vi "SubVI_ReadMatMask_001.vi"(0 "in IMG":bool[][](array[boolean])) -> (1 "Input current":i32[](array[numeric]), 2 "#iter":i32)   [LabVIEW 2018]
uses:
  <vilib>/Analysis/baseanly.llb/Real Dot Product.vi
  <vilib>/Analysis/NI_AALBase.lvlib
panel:
  out "mask":i16[][](array[numeric])
  out "in IMG":i16[][](array[numeric])
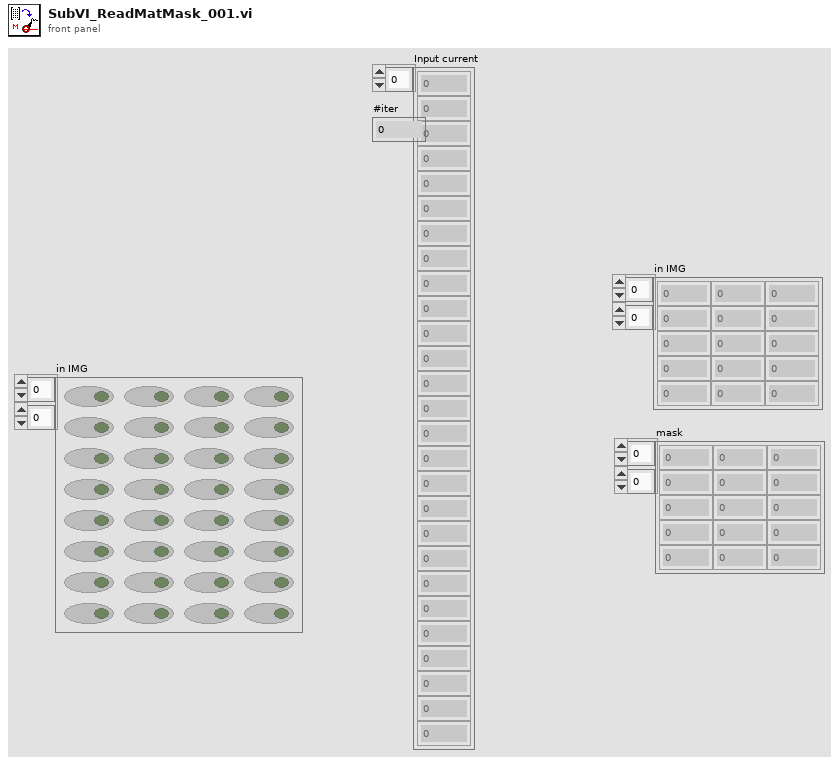
[diagram p1: front panel]
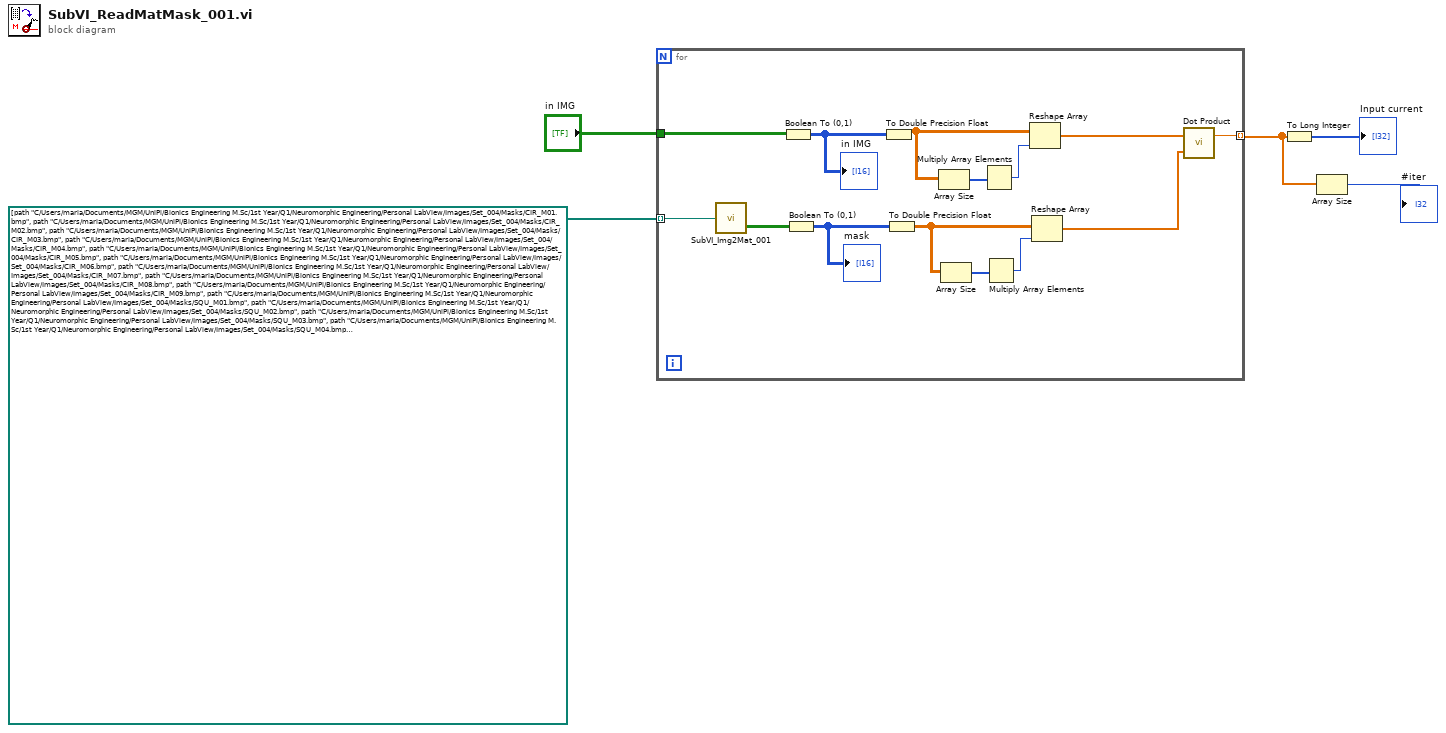
[diagram p0: block diagram]
diagram:
  n1 = for {
    tunnel: [w9] -> w2 mode=indexing
    tunnel: path[] [path "C:/Users/maria/Documents/MGM/UniPi/Bionics Engineering M.Sc/1st Year/Q1/Neuromorphic Engineering/Personal LabView/Images/Set_004/Masks/CIR_M01.bmp", path "C:/Users/maria/Documents/MGM/UniPi/Bionics Engineering M.Sc/1st Year/Q1/Neuromorphic Engineering/Personal LabView/Images/Set_004/Masks/CIR_M02.bmp", path "C:/Users/maria/Documents/MGM/UniPi/Bionics Engineering M.Sc/1st Year/Q1/Neuromorphic Engineering/Personal LabView/Images/Set_004/Masks/CIR_M03.bmp", path "C:/Users/maria/Documents/MGM/UniPi/Bionics Engineering M.Sc/1st Year/Q1/Neuromorphic Engineering/Personal LabView/Images/Set_004/Masks/CIR_M04.bmp", path "C:/Users/maria/Documents/MGM/UniPi/Bionics Engineering M.Sc/1st Year/Q1/Neuromorphic Engineering/Personal LabView/Images/Set_004/Masks/CIR_M05.bmp", path "C:/Users/maria/Documents/MGM/UniPi/Bionics Engineering M.Sc/1st Year/Q1/Neuromorphic Engineering/Personal LabView/Images/Set_004/Masks/CIR_M06.bmp", path "C:/Users/maria/Documents/MGM/UniPi/Bionics Engineering M.Sc/1st Year/Q1/Neuromorphic Engineering/Personal LabView/Images/Set_004/Masks/CIR_M07.bmp", path "C:/Users/maria/Documents/MGM/UniPi/Bionics Engineering M.Sc/1st Year/Q1/Neuromorphic Engineering/Personal LabView/Images/Set_004/Masks/CIR_M08.bmp", path "C:/Users/maria/Documents/MGM/UniPi/Bionics Engineering M.Sc/1st Year/Q1/Neuromorphic Engineering/Personal LabView/Images/Set_004/Masks/CIR_M09.bmp", path "C:/Users/maria/Documents/MGM/UniPi/Bionics Engineering M.Sc/1st Year/Q1/Neuromorphic Engineering/Personal LabView/Images/Set_004/Masks/SQU_M01.bmp", path "C:/Users/maria/Documents/MGM/UniPi/Bionics Engineering M.Sc/1st Year/Q1/Neuromorphic Engineering/Personal LabView/Images/Set_004/Masks/SQU_M02.bmp", path "C:/Users/maria/Documents/MGM/UniPi/Bionics Engineering M.Sc/1st Year/Q1/Neuromorphic Engineering/Personal LabView/Images/Set_004/Masks/SQU_M03.bmp", path "C:/Users/maria/Documents/MGM/UniPi/Bionics Engineering M.Sc/1st Year/Q1/Neuromorphic Engineering/Personal LabView/Images/Set_004/Masks/SQU_M04.bmp", path "C:/Users/maria/Documents/MGM/UniPi/Bionics Engineering M.Sc/1st Year/Q1/Neuromorphic Engineering/Personal LabView/Images/Set_004/Masks/SQU_M05.bmp", path "C:/Users/maria/Documents/MGM/UniPi/Bionics Engineering M.Sc/1st Year/Q1/Neuromorphic Engineering/Personal LabView/Images/Set_004/Masks/SQU_M06.bmp", path "C:/Users/maria/Documents/MGM/UniPi/Bionics Engineering M.Sc/1st Year/Q1/Neuromorphic Engineering/Personal LabView/Images/Set_004/Masks/SQU_M07.bmp", path "C:/Users/maria/Documents/MGM/UniPi/Bionics Engineering M.Sc/1st Year/Q1/Neuromorphic Engineering/Personal LabView/Images/Set_004/Masks/SQU_M08.bmp", path "C:/Users/maria/Documents/MGM/UniPi/Bionics Engineering M.Sc/1st Year/Q1/Neuromorphic Engineering/Personal LabView/Images/Set_004/Masks/SQU_M09.bmp", path "C:/Users/maria/Documents/MGM/UniPi/Bionics Engineering M.Sc/1st Year/Q1/Neuromorphic Engineering/Personal LabView/Images/Set_004/Masks/TRI_M01.bmp", path "C:/Users/maria/Documents/MGM/UniPi/Bionics Engineering M.Sc/1st Year/Q1/Neuromorphic Engineering/Personal LabView/Images/Set_004/Masks/TRI_M02.bmp", path "C:/Users/maria/Documents/MGM/UniPi/Bionics Engineering M.Sc/1st Year/Q1/Neuromorphic Engineering/Personal LabView/Images/Set_004/Masks/TRI_M03.bmp", path "C:/Users/maria/Documents/MGM/UniPi/Bionics Engineering M.Sc/1st Year/Q1/Neuromorphic Engineering/Personal LabView/Images/Set_004/Masks/TRI_M04.bmp", path "C:/Users/maria/Documents/MGM/UniPi/Bionics Engineering M.Sc/1st Year/Q1/Neuromorphic Engineering/Personal LabView/Images/Set_004/Masks/TRI_M05.bmp", path "C:/Users/maria/Documents/MGM/UniPi/Bionics Engineering M.Sc/1st Year/Q1/Neuromorphic Engineering/Personal LabView/Images/Set_004/Masks/TRI_M06.bmp", path "C:/Users/maria/Documents/MGM/UniPi/Bionics Engineering M.Sc/1st Year/Q1/Neuromorphic Engineering/Personal LabView/Images/Set_004/Masks/TRI_M07.bmp", path "C:/Users/maria/Documents/MGM/UniPi/Bionics Engineering M.Sc/1st Year/Q1/Neuromorphic Engineering/Personal LabView/Images/Set_004/Masks/TRI_M08.bmp", path "C:/Users/maria/Documents/MGM/UniPi/Bionics Engineering M.Sc/1st Year/Q1/Neuromorphic Engineering/Personal LabView/Images/Set_004/Masks/TRI_M09.bmp"] ("Masks (path)") -> [w8] mode=indexing
    tunnel: "in IMG" -> [w6]
    n2 = call "SubVI_Img2Mat_001.vi"("Path"=w8) -> ("1-bit pixmap"=w7:bool[][])  [unwired: 1 out]
    n3 = Boolean To (0,1)(Boolean=w6) -> (0, 1=w19:i16[][])
    "in IMG" <- w19
    n4 = Boolean To (0,1)(Boolean=w7) -> (0, 1=w18:i16[][])
    "mask" <- w18
    n5 = To Double Precision Float(number=w19) -> (double precision float=w17:dbl[][])
    n6 = To Double Precision Float(number=w18) -> (double precision float=w12:dbl[][])
    n7 = Array Size(array=w17) -> (size(s)=w15:i32[])
    n8 = Array Size(array=w12) -> (size(s)=w11:i32[])
    n9 = Multiply Array Elements(1:w15) -> (0:w16:i32)
    n10 = Multiply Array Elements(1:w11) -> (0:w13:i32)
    n11 = Reshape Array(w17, w16) -> (w14:dbl[])
    n12 = Reshape Array(w12, w13) -> (w10:dbl[])
    n13 = call-poly <vilib>:"Dot Product.vi"("Y Vector"=w10, "X Vector"=w14) -> ("X * Y"=w9:dbl)  [unwired: 1 out]
  }
  n14 = To Long Integer(number=w2) -> (32bit integer=→"Input current":i32[])
  n15 = Array Size(array=w2) -> (size(s)=→"#iter":i32)
